vi "Test4B2U.vi"() -> ()   [LabVIEW 2021]
uses:
  <instrlib>/IBM4/Public/IBM4_Read(VN).vi
  <instrlib>/IBM4/Public/IBM4_Read(Ave).vi
  <instrlib>/IBM4/IBM4.lvlib
panel:
  out "Average":dbl=1.85786
  out "array":dbl[](array[numeric])
  in  "Mode":enum16{"DC", "AC"}(ring)
  out "Waveform Graph":dbl[](graph)
  in  "COM resource in":refnum<visa-resource-name>
  out "error out":errorcluster
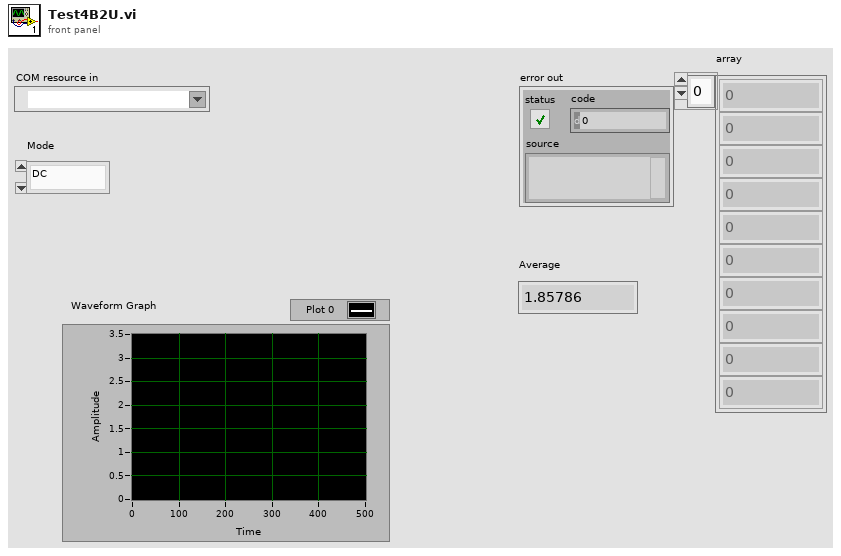
[diagram p1: front panel]
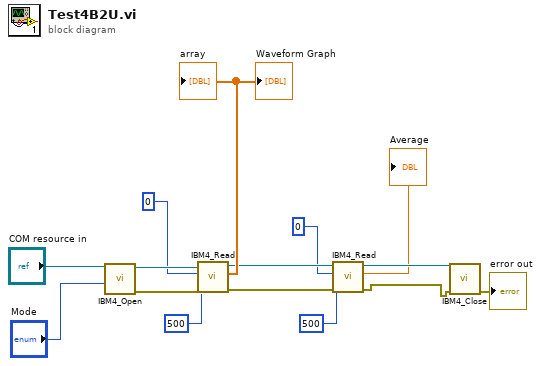
[diagram p0: block diagram]
diagram:
  n1 = call <instrlib>:"IBM4_Open.vi"("Mode"="Mode", "COM Port"="COM resource in") -> ("error out"=w12:errorcluster, "COM resource out"=w13:refnum<visa-resource-name>)  [unwired: 7 in, 1 out]
  n2 = call-poly <instrlib>:"IBM4_Read.vi"("error in"=w12, "Number"=500, "Channel"=0, "COM resource in"=w13) -> ("error out"=w6:errorcluster, "array"=→"Waveform Graph" →"array":dbl[], "COM resource out"=w7:refnum<visa-resource-name>)  [unwired: 5 in]
  n3 = call-poly <instrlib>:"IBM4_Read.vi"("error in"=w6, "Averages"=500, "Channel"=0, "COM resource in"=w7) -> ("error out"=w5:errorcluster, "output"=→"Average":dbl, "COM resource out"=w4:refnum<visa-resource-name>)  [unwired: 5 in]
  n4 = call <instrlib>:"IBM4_Close.vi"("error in"=w5, "COM resource in"=w4) -> ("error out"=→"error out":errorcluster)  [unwired: 9 in]
